vi "sedSpectrometer_getEvent_appliedSettingsMatchStart.vi"(8 "error in (no error)":errorcluster, 11 "logevent_appliedSettingsMatchStart_Ctl":T1) -> (0 "error out":errorcluster, 2 "function return":i32, 3 "logevent_appliedSettingsMatchStart_Ctl out":T1)   [LabVIEW 2016, in "SALLV_sedSpectrometer.lvlib"]
doc: "int sedSpectrometer_shm_getEvent_appliedSettingsMatchStartLV(sedSpectrometer_logevent_appliedSettingsMatchStartLV *logevent_appliedSettingsMatchStart_Ctl );"
uses:
  SALLV_sedSpectrometer.lvlib
  DataTypes/logevent_appliedSettingsMatchStart.ctl
  SALLV_sedSpectrometer.so
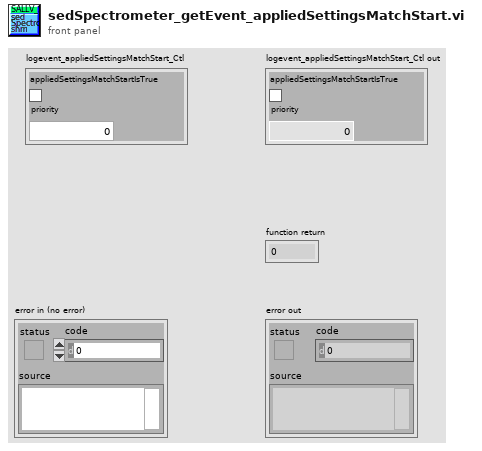
[diagram p1: front panel]
types:
  T1 = typedef "SALLV_sedSpectrometer.lvlib/logevent_appliedSettingsMatchStart.ctl" = cluster{"appliedSettingsMatchStartIsTrue":bool, "priority":i32}
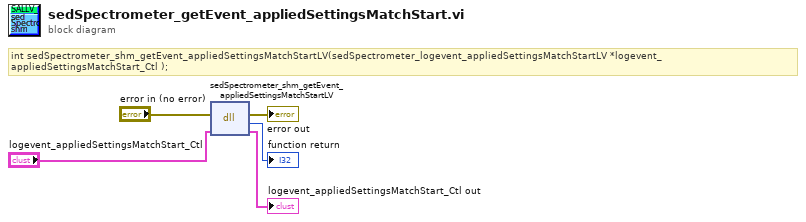
[diagram p0: block diagram]
diagram:
  # "int sedSpectrometer_shm_getEvent_appliedSettingsMatchStartLV(sedSpectrometer_logevent_appliedSettingsMatchStartLV *logevent_appliedSettingsMatchStart_Ctl );"
  n1 = dll-call lib="home/harini/TCS/ts_sallv_sedSpectrometer_371/SALLV_sedSpectrometer.*" fn="sedSpectrometer_shm_getEvent_appliedSettingsMatchStartLV"(error in="error in (no error)", "logevent_appliedSettingsMatchStart_Ctl"="logevent_appliedSettingsMatchStart_Ctl") -> (error out=→"error out":errorcluster, →"function return":i32, "logevent_appliedSettingsMatchStart_Ctl"=→"logevent_appliedSettingsMatchStart_Ctl out":T1)  [unwired: 2 in, 1 out]
